vi "Get Bytes Total.vi"(8 "error in":errorcluster, 11 "Filesystem Statistics in":refnum<class "Filesystem Statistics.lvclass">) -> (0 "error out":errorcluster, 2 "bytes total":u64, 3 "Filesystem Statistics out":refnum<class "Filesystem Statistics.lvclass">)   [LabVIEW 2020, in "NI_SFTP.lvlib" / "Filesystem Statistics.lvclass"]
doc: "Reads the total disk space (in bytes) stored in this Filesystem Statistics object."
uses:
  <vilib>/net/SFTP/Filesystem Statistics/Filesystem Statistics.lvclass
  <vilib>/net/SFTP/Filesystem Statistics/Filesystem Statistics.lvclass/Filesystem Statistics.ctl
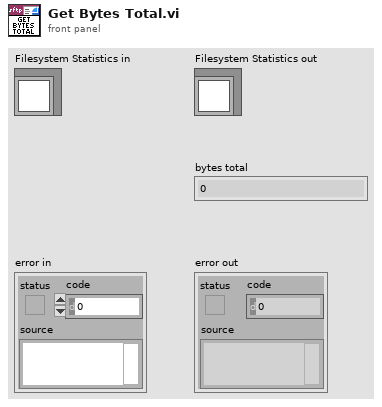
[diagram p1: front panel]
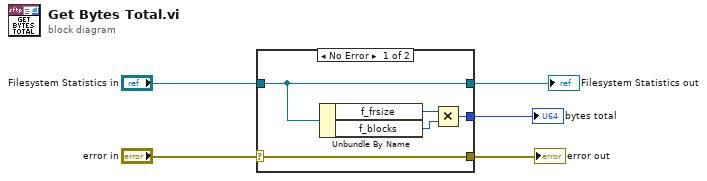
[diagram p0: block diagram]
diagram:
  n1 = case shown="No Error" "error in" {
    selector: "error in" -> [w10 w12]
    tunnel: [w10 w12] -> w2
    tunnel: [w9 w11] -> w3
    tunnel: "Filesystem Statistics in" -> [w9 w11]
    tunnel: [w6 _] -> w1
    frame No Error {
      n2 = Unbundle By Name(w9) -> ("f_frsize"=w8:u64, "f_blocks"=w7:u64)
      n3 = Multiply(x=w8, y=w7) -> (x*y=w6:u64)
    }
    frame Error {
    }
  }
  "error out" <- w2
  "Filesystem Statistics out" <- w3
  "bytes total" <- w1
